vi "niScope Multi Fetch Array Measurement.vi"(0 "instrument handle":refnum<k15>, 1 "timeout":dbl=5.0 format="%.2f", 5 "channels":string="0", 7 "array measurement":T2=4000 items=["None"=4000, "Last Acq. Histogram"=4001, "Multi Acq. Voltage Histogram"=4004, "Multi Acq. Time Histogram"=4005, "Multi Acq. Average"=4016, "Polynomial Interpolation"=4011, "Array Integral"=4006, "Derivative"=4007, "Inverse"=4008, "Multiply Channels"=4012, "Add Channels"=4013, "Subtract Channels"=4014, "Divide Channels"=4015, "Array Offset"=4025, "Array Gain"=4026, "Hanning Window"=4009, "Flat Top Window"=4010, "Hamming Window"=4020, "Triangle Window"=4023, "Blackman Window"=4024, "FIR Windowed Filter"=4021, "Bessel IIR Filter"=4022, "Butterworth IIR Filter"=4017, "Chebyshev IIR Filter"=4018, "FFT Phase Spectrum"=4002, "FFT Amp. Spectrum (Volts RMS)"=4003, "FFT Amp. Spectrum (dB)"=4019], 11 "error in":errorcluster, 12 "meas waveform size":i32=-1) -> (4 "instrument handle out":refnum<k15>, 6 "wfm info":T1(array[cluster]) {"reserved2" format="%.2f"; "reserved1" format="%.2f"; "offset" format="%^.3e"; "gain" format="%^.3e"; "xIncrement" format="%^.3e"; "relativeInitialX" format="%^.3e"; "absoluteInitialX" format="%^.3e"}, 10 "wfm":dbl[][](array[numeric]) format="%.2f", 15 "error out":errorcluster)   [LabVIEW 2013]
doc: "Obtains a waveform from the digitizer and returns the specified measurement voltage data. Unlike the Measurement 1D DBL instance of the niScope Fetch Measurement VI, the Measurement 2D DBL instance can fetch data from multiple channels and records."
uses:
  <instrlib>/niScope/Controls/niScope array measurement.ctl
  niScope_32.dll
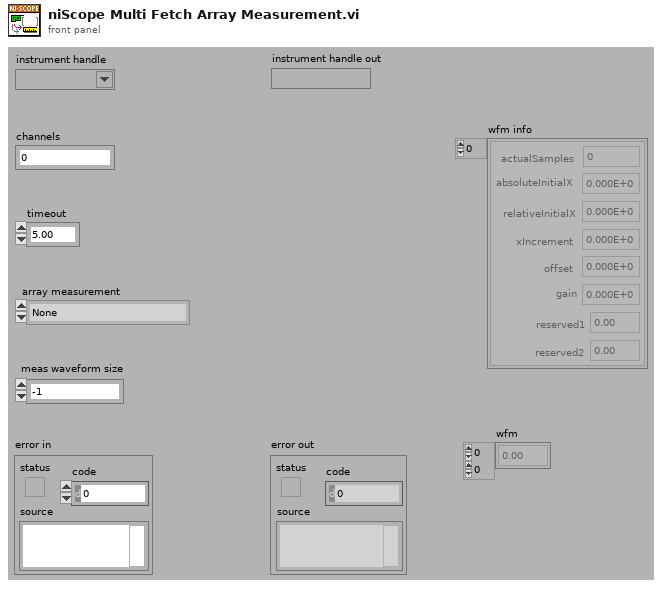
[diagram p1: front panel]
types:
  T1 = cluster{"actualSamples":i32, "absoluteInitialX":dbl, "relativeInitialX":dbl, "xIncrement":dbl, "offset":dbl, "gain":dbl, "reserved1":dbl, "reserved2":dbl}[]
  T2 = typedef "niScope array measurement.ctl" = i32
  T3 = cluster{"Element Data":i32, "Element Data":dbl, "Element Data":dbl, "Element Data":dbl, "Element Data":dbl, "Element Data":dbl, "Element Data":dbl, "Element Data":dbl}
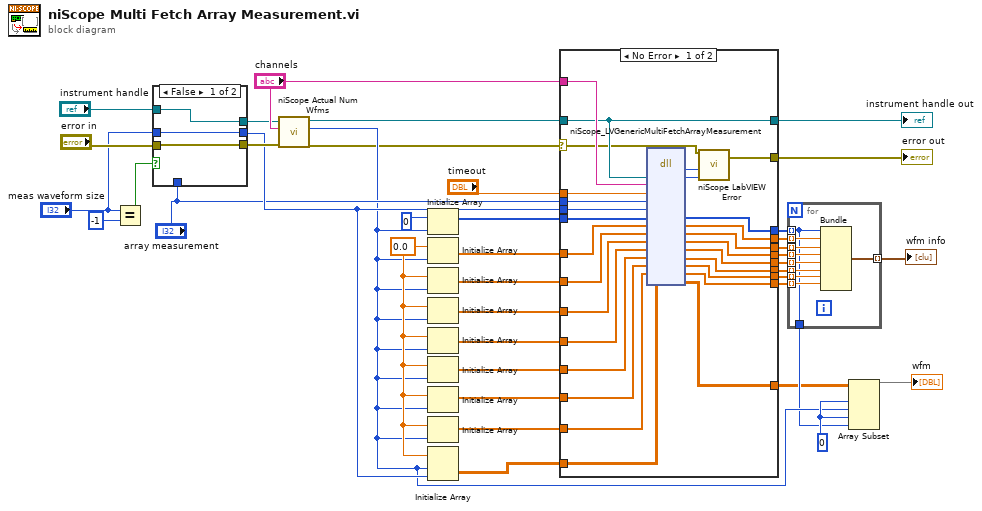
[diagram p0: block diagram]
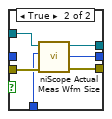
[diagram p3: hidden frame]
diagram:
  w6 = 0 ("Array Index")
  w15 = 0.0 ("Element Data")
  n1 = Equal?(x="meas waveform size", y=-1) -> (x = y?=w37:bool)
  n2 = case shown="False" w37 {
    tunnel: [w43 w49] -> w36
    tunnel: "error in" -> [w43 w48]
    tunnel: "instrument handle" -> [w42 w47]
    tunnel: [w42 w46] -> w33
    tunnel: [w41 w45] -> w31
    tunnel: "meas waveform size" -> [w41 _]
    tunnel: "array measurement" -> [_ w44]
    frame False {
    }
    frame True {
      n3 = call <instrlib>:"niScope Actual Meas Wfm Size.vi"("error in"=w48, "arrayMeasFunction"=w44, "instrument handle"=w47) -> ("error out"=w49:errorcluster, "meas wfm size"=w45:i32, "instrument handle out"=w46:refnum<k15>)  [unwired: 6 in]
    }
  }
  n4 = call <instrlib>:"niScope Actual Num Wfms.vi"("error in"=w36, "channels"="channels", "instrument handle"=w33) -> ("error out"=w1:errorcluster, "actual num wfms"=w5:i32, "instrument handle out"=w8:refnum<k15>)  [unwired: 6 in]
  n5 = Initialize Array(0 ("Element Data"), w5) -> (w10:i32[])
  n6 = Initialize Array(w15, w5) -> (w25:dbl[])
  n7 = Initialize Array(w15, w5) -> (w26:dbl[])
  n8 = Initialize Array(w15, w5) -> (w27:dbl[])
  n9 = Initialize Array(w15, w5) -> (w28:dbl[])
  n10 = Initialize Array(w15, w5) -> (w16:dbl[])
  n11 = Initialize Array(w15, w5) -> (w14:dbl[])
  n12 = Initialize Array(w15, w5) -> (w13:dbl[])
  n13 = Initialize Array(w15, w5, w31) -> (w17:dbl[][])
  n14 = case shown="No Error" w1 {
    selector: w1 -> [w50 w77]
    tunnel: [w76 w77] -> w40
    tunnel: "channels" -> [w75 _]
    tunnel: w31 -> [w74 _]
    tunnel: w8 -> [w51 w78]
    tunnel: w28 -> [w71 w83]
    tunnel: w27 -> [w70 w82]
    tunnel: w26 -> [w69 w81]
    tunnel: w25 -> [w68 w80]
    tunnel: "timeout" -> [w66 _]
    tunnel: [w65 w84] -> w23
    tunnel: [w64 w83] -> w22
    tunnel: [w63 w82] -> w21
    tunnel: [w62 w81] -> w20
    tunnel: [w61 w80] -> w19
    tunnel: [w60 w79] -> w18
    tunnel: "array measurement" -> [w59 _]
    tunnel: w17 -> [w58 w87]
    tunnel: w16 -> [w57 w84]
    tunnel: w14 -> [w56 w85]
    tunnel: w13 -> [w55 w86]
    tunnel: [w54 w85] -> w12
    tunnel: [w53 w86] -> w11
    tunnel: [w52 w87] -> w3
    tunnel: w10 -> [w67 w79]
    tunnel: [w51 w78] -> w7
    frame No Error {
      n15 = dll-call lib="niScope_*.*" fn="niScope_LVGenericMultiFetchArrayMeasurement"("instrument handle"=w51, "channelList"=w75, "timeout"=w66, "arrayMeasFunction"=w59, "measWfmSize"=w74, "actualSamples"=w67, "absoluteInitialX"=w68, "relativeInitialX"=w69, "xIncrement"=w70, "offset"=w71, "gain"=w57, "reserved1"=w56, "reserved2"=w55, "measWfm"=w58) -> ("status"=w73:i32, "instrument handle"=w72:u32, "actualSamples"=w60:i32[], "absoluteInitialX"=w61:dbl[], "relativeInitialX"=w62:dbl[], "xIncrement"=w63:dbl[], "offset"=w64:dbl[], "gain"=w65:dbl[], "reserved1"=w54:dbl[], "reserved2"=w53:dbl[], "measWfm"=w52:dbl[][])  [unwired: 7 in, 2 out]
      n16 = call <instrlib>:"niScope LabVIEW Error.vi"("instrument handle"=w72, "niScope error code (0)"=w73, "error in (no error)"=w50) -> ("error out"=w76:errorcluster)  [unwired: 2 in]
    }
    frame Error {
    }
  }
  "error out" <- w40
  "instrument handle out" <- w7
  n17 = for {
    tunnel: w18 -> [w88] mode=indexing
    tunnel: w19 -> [w96] mode=indexing
    tunnel: w20 -> [w93] mode=indexing
    tunnel: w21 -> [w92] mode=indexing
    tunnel: w22 -> [w95] mode=indexing
    tunnel: w23 -> [w94] mode=indexing
    tunnel: [w91] -> w30 mode=indexing
    tunnel: w12 -> [w90] mode=indexing
    tunnel: w11 -> [w89] mode=indexing
    tunnel: [w88] -> w4
    n18 = Bundle("Element Data"=w88, "Element Data"=w96, "Element Data"=w93, "Element Data"=w92, "Element Data"=w95, "Element Data"=w94, "Element Data"=w90, "Element Data"=w89) -> (w91:T3)  [unwired: 1 in]
  }
  "wfm info" <- w30
  n19 = Array Subset(array=w3, index (row)=w6, length (row)=w5, index (col)=w6, length (col)=w4) -> (→"wfm":dbl[][])
